vi "CalcDlyTimePFI.vi"(6 "Limits":dbl[][](array[numeric])=[[0.059450168900494, 0.0606065605190911, 0.056793034460449, 0.0377791964132806, 0.0387680244678906, 0.041509529284321, 0.0, 0.0], [0.0543254248656728, 0.0605582232708396, 0.0705532258276927, 0.0403341376210629, 0.0362750710120636, 0.037641124860868, 0.0, 0.0], [0.0542535208152999, 0.0601149006696316, 0.057100190511556, 0.0286705153398605, 0.0306659503421681, 0.0318434771124804, 0.0, 0.0], [0.0539806772823237, 0.060111916581221, 0.0568149701475802, 0.0287477348403936, 0.030687681069202, 0.0318140233011936, 0.0, 0.0], [0.0574739206185427, 0.0628177175852463, 0.0608742935192014, 0.0507031710323209, 0.0492196025001063, 0.0512494967622953, 0.0, 0.0], [0.0573743399751993, 0.0636926206100454, 0.0626583117825458, 0.0369031527657219, 0.0385466857090226, 0.0400368175447213, 0.0, 0.0], [0.0831820808794742, 0.0842623844587226, 0.088262229564689, 0.0667743079383481, 0.0680308099651913, 0.0679787518894359, 0.0, 0.0], [0.0541037185786453, 0.0597178605956032, 0.0641248041876747, 0.0281653525639868, 0.0301909812864416, 0.0304719216326717, 0.0, 0.0], [0.0564462783136314, 0.0600214622402702, 0.0759912985981658, 0.0281162118220652, 0.0301892901163339, 0.0303638978137465, 0.0, 0.0], [0.0540653703792215, 0.0598738420777627, 0.0612858805251609, 0.0282196395706911, 0.0301950277548319, 0.0310242020330342, 0.0, 0.0], [0.056709051486753, 0.0602058925674664, 0.0806981932623049, 0.0281451428430134, 0.0302542048015808, 0.0304691904137436, 0.0, 0.0]], 11 "Results":dbl[][][](array[numeric])) -> (3 "PFI":string[][](array[string]))   [LabVIEW 2014]
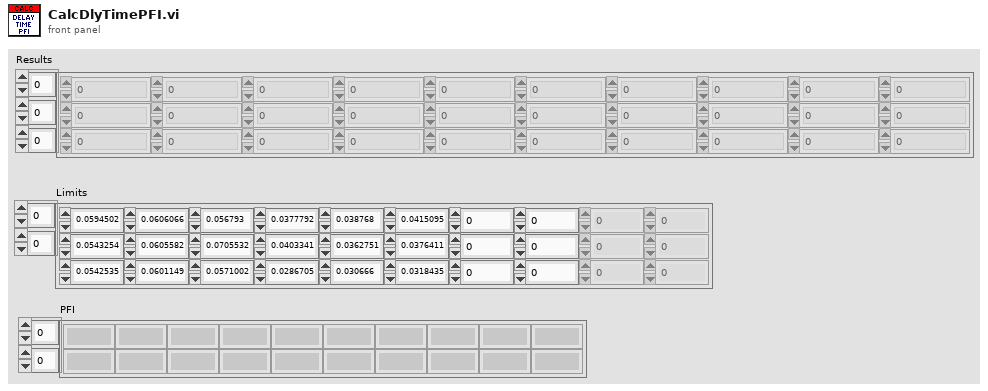
[diagram p1: front panel]
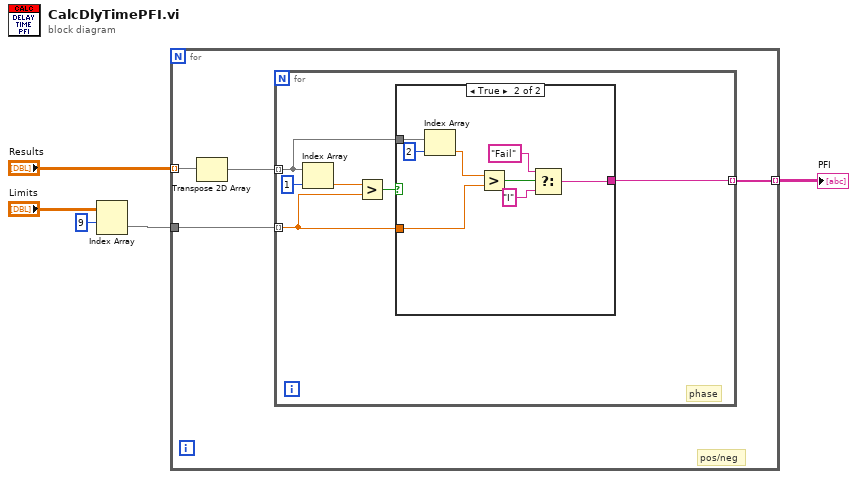
[diagram p0: block diagram]
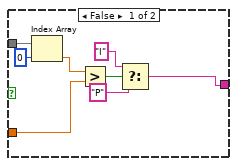
[diagram p2: hidden frame]
diagram:
  n1 = Index Array(array="Limits", index (row)=9) -> (element=w2:dbl[])  [unwired: 1 in]
  n2 = for {
    tunnel: "Results" -> [w8] mode=indexing
    tunnel: w2 -> [w9]
    tunnel: [w6] -> w1 mode=indexing
    # "pos/neg"
    n3 = Transpose 2D Array(2D array=w8) -> (transposed array=w7:dbl[][])
    n4 = for {
      tunnel: w9 -> [w11] mode=indexing
      tunnel: w7 -> [w12] mode=indexing
      tunnel: [w10] -> w6 mode=indexing
      # "phase"
      n5 = Index Array(array=w12, index=1) -> (element=w14:dbl)
      n6 = Greater?(x=w14, y=w11) -> (0:w13:bool)
      n7 = case shown="True" w13 {
        tunnel: w12 -> [w23 w31]
        tunnel: w11 -> [w20 w28]
        tunnel: [w18 w24] -> w10
        frame False {
          n8 = Index Array(array=w23, index=0) -> (element=w21:dbl)
          n9 = Greater?(x=w21, y=w20) -> (0:w19:bool)
          n10 = Select(t="I", s=w19, f="P") -> (s? t:f=w18:string)
        }
        frame True {
          n11 = Index Array(array=w31, index=2) -> (element=w29:dbl)
          n12 = Greater?(x=w29, y=w28) -> (0:w27:bool)
          n13 = Select(t="Fail", s=w27, f="I") -> (s? t:f=w24:string)
        }
      }
    }
  }
  "PFI" <- w1
